vi "MAIN_PECT.vi"() -> ()   [LabVIEW 2018]
uses:
  <vilib>/DAQmx/read.llb/DAQmx Read (Analog 2D DBL NChan NSamp).vi
  <vilib>/Analysis/baseanly.llb/Mean (DBL).vi
  <vilib>/Instr/_visa.llb/VISA Configure Serial Port (Instr).vi
  <vilib>/DAQmx/create/channels.llb/DAQmx Create Channel (AI-Voltage-Basic).vi
  <vilib>/DAQmx/configure/timing.llb/DAQmx Timing (Sample Clock).vi
  <vilib>/DAQmx/configure/trigger.llb/DAQmx Start Trigger (Digital Edge).vi
  <vilib>/DAQmx/miscellaneous.llb/DAQmx Fill In Error Info.vi
  <resource>/objmgr/daqmx.rc
  <vilib>/Analysis/NI_AALBase.lvlib
  <vilib>/Platform/NI_3dgraph.lvlib
panel:
  out "Enum":T1(ring)=enum."Wait X"
  out "Current  Position (mm)":dbl=34.0
  out "Numeric":dbl=53.0
  in  "3D Surface":refnum<k7>(container)
  out "Feature extraction scan":dbl[](graph)=[0.08283467438816226, 0.08315021104927388, 0.08279539001624267, 0.08264303586690222, 0.08270737694574541, 0.08275255148264649, 0.08273400780940561, 0.08285927976479214, 0.08269226561515775, 0.08297621309518552, 0.08311167850920542, 0.08274828411115004, 0.08283507475884443, 0.08288811917638333, 0.08284021281644091, 0.08265273310686665, 0.082873404050702, 0.08252929871145775, 0.08289438074272544, 0.08328077996201763, 0.082870445586509, 0.08280965226600595, 0.08297444941499994, 0.08288058058223531, 0.08286124313516094, 0.08284469301402564, 0.083066551569298, 0.08282839970840086, 0.08295066176596085, 0.08313066697548752, 0.08296193038583091, 0.08281760657720119, 0.08275185969129775, 0.0830021575495491, 0.08289519151448965, 0.08270942154189498, 0.08314587726689038, 0.08300520769005512, 0.08316588069373743, 0.08268431002182852, 0.08284144737975019, 0.08280888249300979, 0.08277531905033915, 0.08291205402335713, 0.08302780379458881, 0.08284349413031018, 0.08272722568614103, 0.08294041368027252, 0.08290046841469481, 0.08300386096775844, 0.08306896615572697, 0.08269688952804832, 0.08275967850911117, 0.08263417478426685, 0.08279623232481706, 0.08272915933307569, 0.08286824410754713, 0.08291091733726794, 0.0830296712620475, 0.08266577930171704, 0.08258683375256373, 0.08276733860182627, 0.08282634908830305, 0.08298619981585892, 0.0828967582780724, 0.08282850993163872, 0.08273475855683762, 0.082968978472369, 0.0829109484443218, 0.0825587351950988, 0.08283584901550614, 0.08287979050131826, 0.08268241229465044, 0.08277735726888424, 0.08256618170984673, 0.08284253191870816, 0.08275059580850669, 0.08290221877356678, 0.08312313437093057, 0.0831193939376253, 0.08297293429910735, 0.08295049977967987, 0.08297761508701938, 0.08282735150019817, 0.0831591264906493, 0.08295251198394006, 0.08302823676291486, 0.08296307164975165, 0.08249046862995961, 0.08231989615770464, 0.08138645179421407, 0.07945694677113982, 0.07933082551380949, 0.08029170332009304, 0.08139752467180725, 0.08244302749015182, 0.08257548202947437, 0.08253717111330304, 0.0829704375877119, 0.08287075930532974, 0.08268538709012521, 0.08312089775665858, 0.08317847119013734, 0.0830002175397772, 0.082882772850329, 0.08311676213140336, 0.08291783582333187, 0.0829506193255121, 0.08276986520948888, 0.08300046343378967, 0.08275137325508078, 0.08277619485982919, 0.0828156000102155, 0.08269641985397105, 0.08263873798983143, 0.08270377967400899, 0.08291552507873104, 0.08270508332182003, 0.08289923248519893, 0.08282877191228727]
  in  "Cursor":bool=TRUE
  out "Completed":bool
  out "Acquire":bool
  in  "Step X":dbl=0.5
  in  "Freq_Sampling_SizeX_SizeY":dbl[](array[numeric])=[300.0, 100000.0]
  in  "Direction (+)":string="-"
  in  "X - length":dbl=60.0
  in  "Step Y":dbl=0.5
  in  "Y - length":dbl=60.0
  out "Start Pos Y":dbl
  out "Start Pos X":dbl
  in  "Scan":bool=TRUE
  in  "Motor only":bool
  out "Waveform Chart 2":dbl(graph)=0.08264330967693855
  in  "Offset":bool
  in  "Gate 2":dbl=25.0
  in  "Gate 1":dbl
  out "Backdata":dbl
  in  "Backdata":bool
  in  "Frame Avr.":i32=10
  in  "Digital Start Trigger Edge":i32(ring)=10280 caption="Edge" items=["Rising"=10280, "Falling"=10171]
  in  "Digital Start Trigger Source":tag="/Dev3/PFI0" caption="Trigger"
  in  "Move Dis(mm)":dbl=100.0
  out "Y Current.Pos(mm)":dbl=4.5 format="%#_4g"
  in  "COM Y":refnum<visa-resource-name>="COM3"
  in  "Multiplier":dbl=10.0
  in  "Travel per Pulse (mm)":dbl=0.004
  out "X Current.Pos(mm)":dbl=33.356 format="%#_4g"
  in  "Flow control":u16(ring) items=["None", "XON/XOFF", "RTS/CTS", "XON/XOFF & RTS/CTS", "DTR/DSR", "XON/XOFF & DTR/DSR"]
  in  "Stop bits":u16(ring)=10 items=["1.0"=10, "1.5"=15, "2.0"=20]
  in  "Speed (mm/s)":dbl=3.0
  in  "Stop":bool
  in  "Home":bool
  in  "Backward":bool
  in  "Left":bool
  in  "Forward":bool
  in  "Right":bool
  in  "Exit":bool
  in  "Parity":dbl
  in  "Data bits":u16=8 min=5 max=8 step=1
  in  "Baud Rate":u32=9600
  in  "COM X":refnum<visa-resource-name>="COM4"
  out "Waveform Graph 2":dbl[][](graph)=[[0.013601434298277221, 0.08376748657539852, 0.10555538260692392, 0.09988279438437878, 0.10291247214781425, 0.11561133460895198, 0.11364526707076025, 0.1047818478966451, 0.1184476286984939, 0.11196927511842217, 0.10416946617730119, 0.11116350971762164, 0.11264611793148685, 0.10397608257206907, 0.10935859528632208, 0.11171143016114275, 0.11361303649046076, 0.10852059925027957, 0.11586917952203521, 0.1124205037193586, 0.10584545813755739, 0.10919744219139764, 0.11280727102984134, 0.10397608256605081, 0.11080897297082777, 0.111066817844625, 0.11383865080705668, 0.10810160124557855, 0.11316180785941188, 0.11232381178111188, 0.10584545814989085, 0.10997097694527913, 0.11464441610483356, 0.10510415409350957, 0.11271057919576397, 0.11200150570035368, 0.11048666681159183, 0.10774706448063742, 0.11206596695446602, 0.11032551365379104, 0.10336370079032715, 0.10980982388310886, 0.11554687331452282, 0.10855282989125889, 0.1136774976544753, 0.11335519151887692, 0.10945528709246041, 0.10803714001130564, 0.11016436061280914, 0.10926190340085944, 0.09843241667361965, 0.11129243219726545, 0.11802863066881217, 0.10813383190229638, 0.11158250773738898, 0.11773855507696329, 0.10777929514448825, 0.10771483386556273, 0.1119370444031454, 0.1106478198754941, 0.09943156577112659, 0.11448326307988417, 0.11715840405452091, 0.10600661130849598, 0.11264611798894486, 0.11770632446719906, 0.10674791544461082, 0.10723137460757921, 0.11432210997511645, 0.11161473830411259, 0.10133317204675463, 0.11467664676291349, 0.11957570018781452, 0.10558761331160751, 0.10890736659450233, 0.1153212590005039, 0.10700576038234985, 0.10436284984003283, 0.11509564479684438, 0.11661048364039184, 0.10249347419312219, 0.11383865078746372, 0.12057484923885912, 0.10497523162681976, 0.10703799090530461, 0.11480556919139581, 0.10520084593006562, 0.10384716002193348, 0.11419318748956753, 0.1157724876889634, 0.10545869077007768, 0.11522456723740233, 0.12221861059120405, 0.10861729104683968, 0.10439508050894415, 0.11348411399724478, 0.10658676239523164, 0.10703799096366998, 0.11348411394953914, 0.11483779983544758, 0.105748766286294, 0.11364526710593634, 0.12089715535436718, 0.10842390737397982, 0.10358931516306184, 0.11351634464482596, 0.10839167680425396, 0.10974536256547154, 0.11428987936827059, 0.11506341408623584, 0.10433061916843969, 0.11184035263979672, 0.11625594670038104, 0.10439508050888772, 0.10758591145457821, 0.11699725106811235, 0.11097012602935477, 0.11077674228063383, 0.11690055921882556, 0.1119370443655943, 0.10391162120758887, 0.11100235666681757, 0.11377418946627674, 0.10313808654861531, 0.10668345422161463, 0.12063931049392565, 0.11213042817800026, 0.11032551358979706, 0.11748071025092614, 0.11171143006960613, 0.10600661125928526, 0.10723137464977092, 0.11551464274992203, 0.1009141740623463, 0.11000320758245671, 0.12205745752266203, 0.1106800504822431, 0.1088751360032324, 0.12070377174855577, 0.10806937058012958, 0.10568430507660669, 0.10961644014725073, 0.11532125899335136, 0.10084971283493516, 0.1129684241513111, 0.1211872309349945, 0.11055112802413684, 0.10613553370420262, 0.11964016142031346, 0.10674791538099922, 0.10371823751735168, 0.11245273434937711, 0.11722286520589442, 0.10578099696801421, 0.11164696886759451, 0.12228307187689273, 0.11013213004518332, 0.10204224553504146, 0.11673940609854719, 0.10819829306708265, 0.10265462716988191, 0.11470887734845048, 0.12099384718962294, 0.10652230113094655, 0.1138064201020185, 0.12221861065750776, 0.1102610524735794, 0.08334848852242217, -0.058788534635624334, -0.11989779045978155, -0.14017085139642654, -0.1336280352805537, -0.12801990704400926, -0.14600459383486838, -0.13801139971037607, -0.1311462772922099, -0.14107330877412233, -0.14967888479881436, -0.13733455662936145, -0.14065431057136318, -0.14774504739847086, -0.13475610701189997, -0.13156527533589288, -0.14858304359243135, -0.14136338429903875, -0.13079174085124246, -0.14258814791681923, -0.15029126661441775, -0.12972812989040167, -0.14197576622098812, -0.14484429156186746, -0.13362803512777408, -0.13166196732019605, -0.15132264646204385, -0.14171792120587728, -0.13240327180667855, -0.14858304358489416, -0.14671366757571636, -0.1247968448647718, -0.14242699487971355, -0.1427493011356822, -0.13224211836195246, -0.1359808705608181, -0.15035572777198442, -0.14719712698964665, -0.13140412236860619, -0.15103257084729058, -0.14371621972211224, -0.1263116841459282, -0.1403642349991318, -0.1424592254369844, -0.12889013376813427, -0.14191130491799478, -0.14809958426479436, -0.14677812889654474, -0.13111404665168178, -0.15177387515944252, -0.13936508580925389, -0.12669845160863982, -0.1428459928421259, -0.14700374310609157, -0.13037274236425173, -0.1458756714525446, -0.14684259002493194, -0.14361952793272406, -0.13104958540060116, -0.14677812876602267, -0.1381080916109839, -0.13108181602987884, -0.14233030290956655, -0.1491954254599751, -0.1326611164851572, -0.144167448547146, -0.15051688097972826, -0.14023531251808827, -0.12885790319962048, -0.14274930102339384, -0.1415245375090149, -0.13111404663251974, -0.14336168282353604, -0.1502590359852162, -0.13688332796086422, -0.14091215576342137, -0.15112926275912902, -0.14004192882973127, -0.12808436827914507, -0.14181461295870892, -0.1407510025200201, -0.1309206629510732, -0.14339391351034778, -0.15454570867573808, -0.13913947146510475, -0.13817255274502313, -0.15190279768123222, -0.13620648496892968, -0.1339825719914834, -0.14303937657753946, -0.14220138051954856, -0.13330572894558984, -0.14107330876402224, -0.15322425317405103, -0.13527179685661722, -0.13926839391275525, -0.1468425900501376, -0.13765686282695927, -0.13395034137824646, -0.14913096409414178, -0.14220138056245094, -0.13610979309633864, -0.1428459929306679, -0.1514193383764275, -0.13362803506894924, -0.13694778927852186, -0.14529552018613665, -0.13627094604099171, -0.13662548295342475, -0.14664920627251926, -0.14703597378395564, -0.13720563421577722, -0.14407075652821602, -0.14787396992634924, -0.13565856431412787, -0.1359808705794155, -0.1445864464810054, -0.1380436302301929, -0.14162122931720006, -0.14307160730830817, -0.1510970321115987, -0.1368188666778612, -0.14323276036380136, -0.14626243883029288, -0.13652879115001798, -0.13301565343259897, -0.14681035935072898, -0.1381080914941658, -0.14123446183340477, -0.14071877196186522, -0.1513871077424996, -0.13543294994218183, -0.14213691925180744], [0.5037481552143733, 0.4782859739390544, 0.5250203570724526, 0.49504589076072747, 0.4966574212176529, 0.48118672878275026, 0.534367233585223, 0.4808644226891975, 0.5098719709209371, 0.5150288683453328, 0.5095496648315279, 0.477963667845071, 0.5263095814212335, 0.4956905029436372, 0.49407897248601346, 0.4808644226891975, 0.5179296231414922, 0.483442871436285, 0.5024589308529928, 0.5166403987880918, 0.5130950318125386, 0.48569901408749055, 0.5188965414060729, 0.5024589308529928, 0.49053360547513025, 0.4911782176593487, 0.5056819917550686, 0.48569901408749055, 0.5018143186720267, 0.5134173379014503, 0.5085827465630276, 0.4937566663943488, 0.5140619500791384, 0.5063266039349343, 0.49085591156726294, 0.503425849124097, 0.503425849124097, 0.4889220750137619, 0.5002027882188058, 0.5121281135455329, 0.5014920125814748, 0.5005250943095422, 0.510194277010301, 0.5105165830996194, 0.4869882384585658, 0.5140619500791384, 0.5018143186720267, 0.49407897248601346, 0.4966574212176529, 0.5185742353179239, 0.4934343603026375, 0.5043927673947882, 0.5031035430337749, 0.5098719709209371, 0.4892443811061296, 0.5188965414060729, 0.5027812369434068, 0.4998804821280232, 0.4985912577644308, 0.5304995605499158, 0.4882774628288851, 0.5011697064908767, 0.5060042978450243, 0.5050373795750199, 0.48215364706312236, 0.5240534388104038, 0.5005250943095422, 0.5014920125814748, 0.49085591156726294, 0.5424248857221113, 0.48795515673637607, 0.5037481552143733, 0.504715073484927, 0.5085827465630276, 0.47860828003298983, 0.523086520547957, 0.5008474004002325, 0.5014920125814748, 0.480542116595597, 0.541457967467102, 0.4892443811061296, 0.5002027882188058, 0.5105165830996194, 0.5130950318125386, 0.47602983128016196, 0.5234088266354835, 0.5040704613046038, 0.4985912577644308, 0.47538521909147413, 0.5308218666364309, 0.4892443811061296, 0.5018143186720267, 0.5118058074564408, 0.5234088266354835, 0.47506291299705794, 0.5205080718461484, 0.510194277010301, 0.49472358466920274, 0.4776413617510396, 0.5166403987880918, 0.4892443811061296, 0.4995581760371945, 0.5118058074564408, 0.5243757448977976, 0.4895666871984503, 0.5150288683453328, 0.5166403987880918, 0.49021129938295055, 0.4892443811061296, 0.5095496648315279, 0.49053360547513025, 0.49504589076072747, 0.5150288683453328, 0.5159957866111228, 0.4969797273088985, 0.5072935222043906, 0.5179296231414922, 0.4911782176593487, 0.4989135638553983, 0.5092273587420731, 0.4969797273088985, 0.4937566663943488, 0.5124504196345799, 0.5095496648315279, 0.4969797273088985, 0.5037481552143733, 0.5179296231414922, 0.4921451359353248, 0.510194277010301, 0.5072935222043906, 0.5040704613046038, 0.4924674420272231, 0.5243757448977976, 0.4989135638553983, 0.4973020334000977, 0.5005250943095422, 0.516962704876509, 0.48795515673637607, 0.516962704876509, 0.5076158282941181, 0.5060042978450243, 0.4953681968522056, 0.5363010701005323, 0.4976243394912505, 0.4918228298433796, 0.5011697064908767, 0.5159957866111228, 0.47860828003298983, 0.5201857657582224, 0.5069712161146175, 0.5056819917550686, 0.48569901408749055, 0.5411356613820134, 0.49504589076072747, 0.49826895167341706, 0.5037481552143733, 0.5185742353179239, 0.47602983128016196, 0.5227642144603862, 0.5082604404734367, 0.5040704613046038, 0.4718398520502395, 0.5356564579289357, 0.49407897248601346, 0.4969797273088985, 0.5072935222043906, 0.5275988057693101, -0.5192517469977762, -0.4812195963717544, -0.4818642090794271, -0.49959105873960724, -0.5337555337266507, -0.47348424391910443, -0.5070041050757489, -0.5031364287179863, -0.48605419169165304, -0.46832734232432, -0.5169956024191665, -0.48218651543345337, -0.4818642090794271, -0.5002356714617954, -0.5256978744002724, -0.48315343449629206, -0.5070041050757489, -0.5073264114397315, -0.48412035356027106, -0.47090579311768965, -0.5060371859845731, -0.487343417115113, -0.4763850010803293, -0.504425654168518, -0.5115163941832249, -0.4886326425406057, -0.5012025905460384, -0.5140948451131326, -0.4847649662702243, -0.4802526773111943, -0.504425654168518, -0.4937895442629384, -0.4776742264885969, -0.5047479605314721, -0.5002356714617954, -0.4895995616110602, -0.49540107605786016, -0.5131279260134487, -0.48315343449629206, -0.486698804403129, -0.5053925732577655, -0.4989464460179313, -0.47574038837695243, -0.5070041050757489, -0.4950787696986205, -0.48605419169165304, -0.49056648068265996, -0.5157063769485245, -0.46993887406923396, -0.4944341569805242, -0.5095825559912142, -0.5037810414429954, -0.47509577567408007, -0.5157063769485245, -0.4886326425406057, -0.48605419169165304, -0.4937895442629384, -0.5182848278918804, -0.4593027646106859, -0.5008802841844959, -0.5076487178038427, -0.4999133651006372, -0.47864114554612325, -0.5173179087871507, -0.4883103361840418, -0.48927725525411486, -0.4947564633395085, -0.5282763253758406, -0.46284813441505984, -0.49959105873960724, -0.5050702668945546, -0.49797952693637737, -0.47058348676807876, -0.5179625215235075, -0.4883103361840418, -0.4889549488972967, -0.49217801247120607, -0.5373009038561416, -0.4715504058172886, -0.49959105873960724, -0.5063594923481698, -0.49121109339769625, -0.4673604232788777, -0.5153840705811875, -0.48992186796813286, -0.4895995616110602, -0.4950787696986205, -0.5340778401014041, -0.486698804403129, -0.4989464460179313, -0.5070041050757489, -0.4918557061132421, -0.46510427884390065, -0.5099048623562269, -0.49701260785597473, -0.48379804720548464, -0.4989464460179313, -0.5247309552865832, -0.49056648068265996, -0.4950787696986205, -0.5082933305324514, -0.49411185062166746, -0.4715504058172886, -0.5053925732577655, -0.5021695096314351, -0.48347574085082495, -0.49797952693637737, -0.5111940878175674, -0.4944341569805242, -0.48992186796813286, -0.5082933305324514, -0.4973349142159811, -0.4818642090794271, -0.5060371859845731, -0.5082933305324514, -0.48154190272552744, -0.4999133651006372, -0.5024918159934906, -0.48927725525411486, -0.4895995616110602, -0.5105494750866392, -0.4889549488972967, -0.4934672379043369, -0.5041033478056925, -0.5082933305324514, -0.48702111075905746, -0.49926875237870527, -0.49862413965728536, -0.49153339975540544, -0.4854095789806849, -0.5079710241680827, -0.4879880298276051, -0.49411185062166746]]
  in  "length":i32
  in  "Start index":i32
  in  "Path":path
  in  "Name File":string
  in  "SAVE ?":bool
  in  "Number of Samples":i32=400
  in  "Sample Rate":dbl=100000.0
  in  "Sample Clock Source":tag="OnboardClock"
  in  "Terminal Configuration":i32(ring)=10083 items=["default"=-1, "RSE"=10083, "NRSE"=10078, "Differential"=10106, "Pseudodifferential"=12529]
  in  "Max Voltage":dbl=10.0
  in  "Min Voltage":dbl=-10.0
  in  "Physical Channel":tag="Dev3/ai1:2"
  out "Actual Sample Rate":dbl=100000.0 format="%0.2f"
  # "Graph"
  # "Channel Settings"
  # "Control Program"
  # "Timing Settings"
  # "Saving Data Settings"
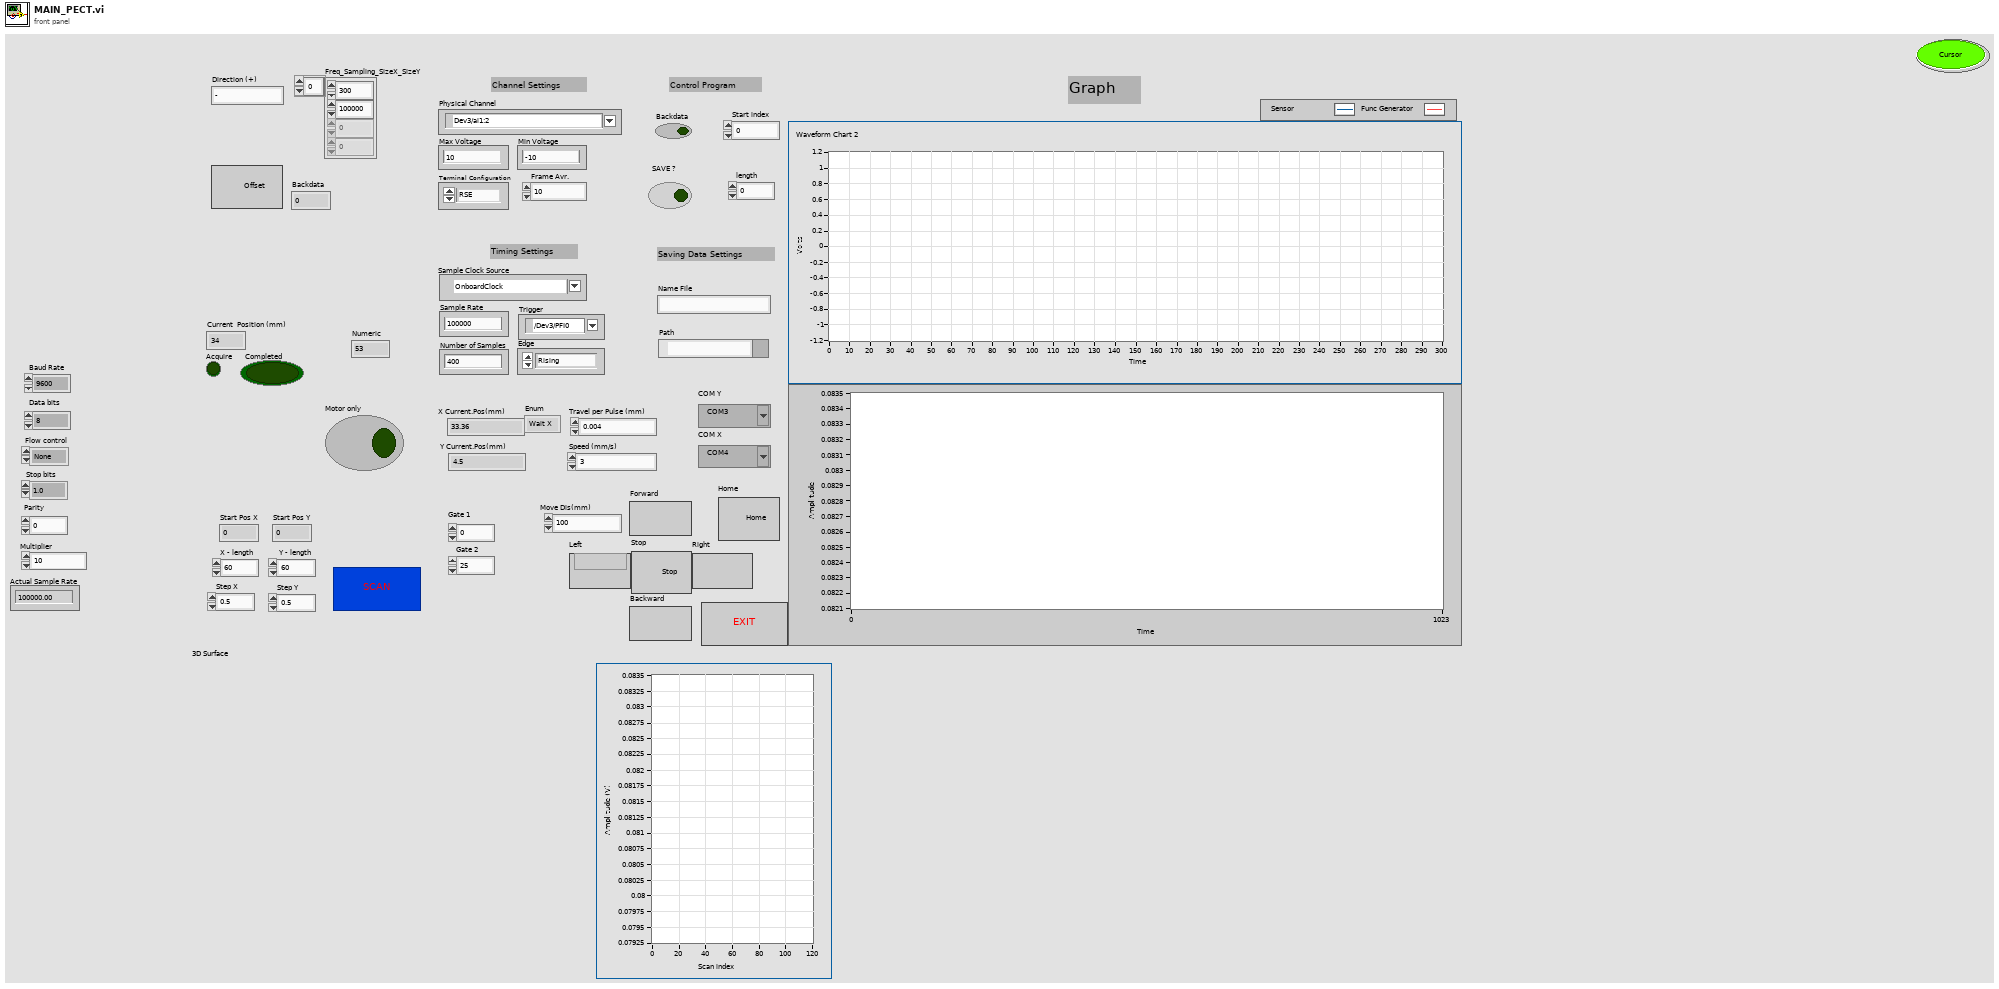
[diagram p1: front panel]
types:
  T1 = enum16{"No Scan", "Move X", "Wait X", "Move Y", "Wait Y"}
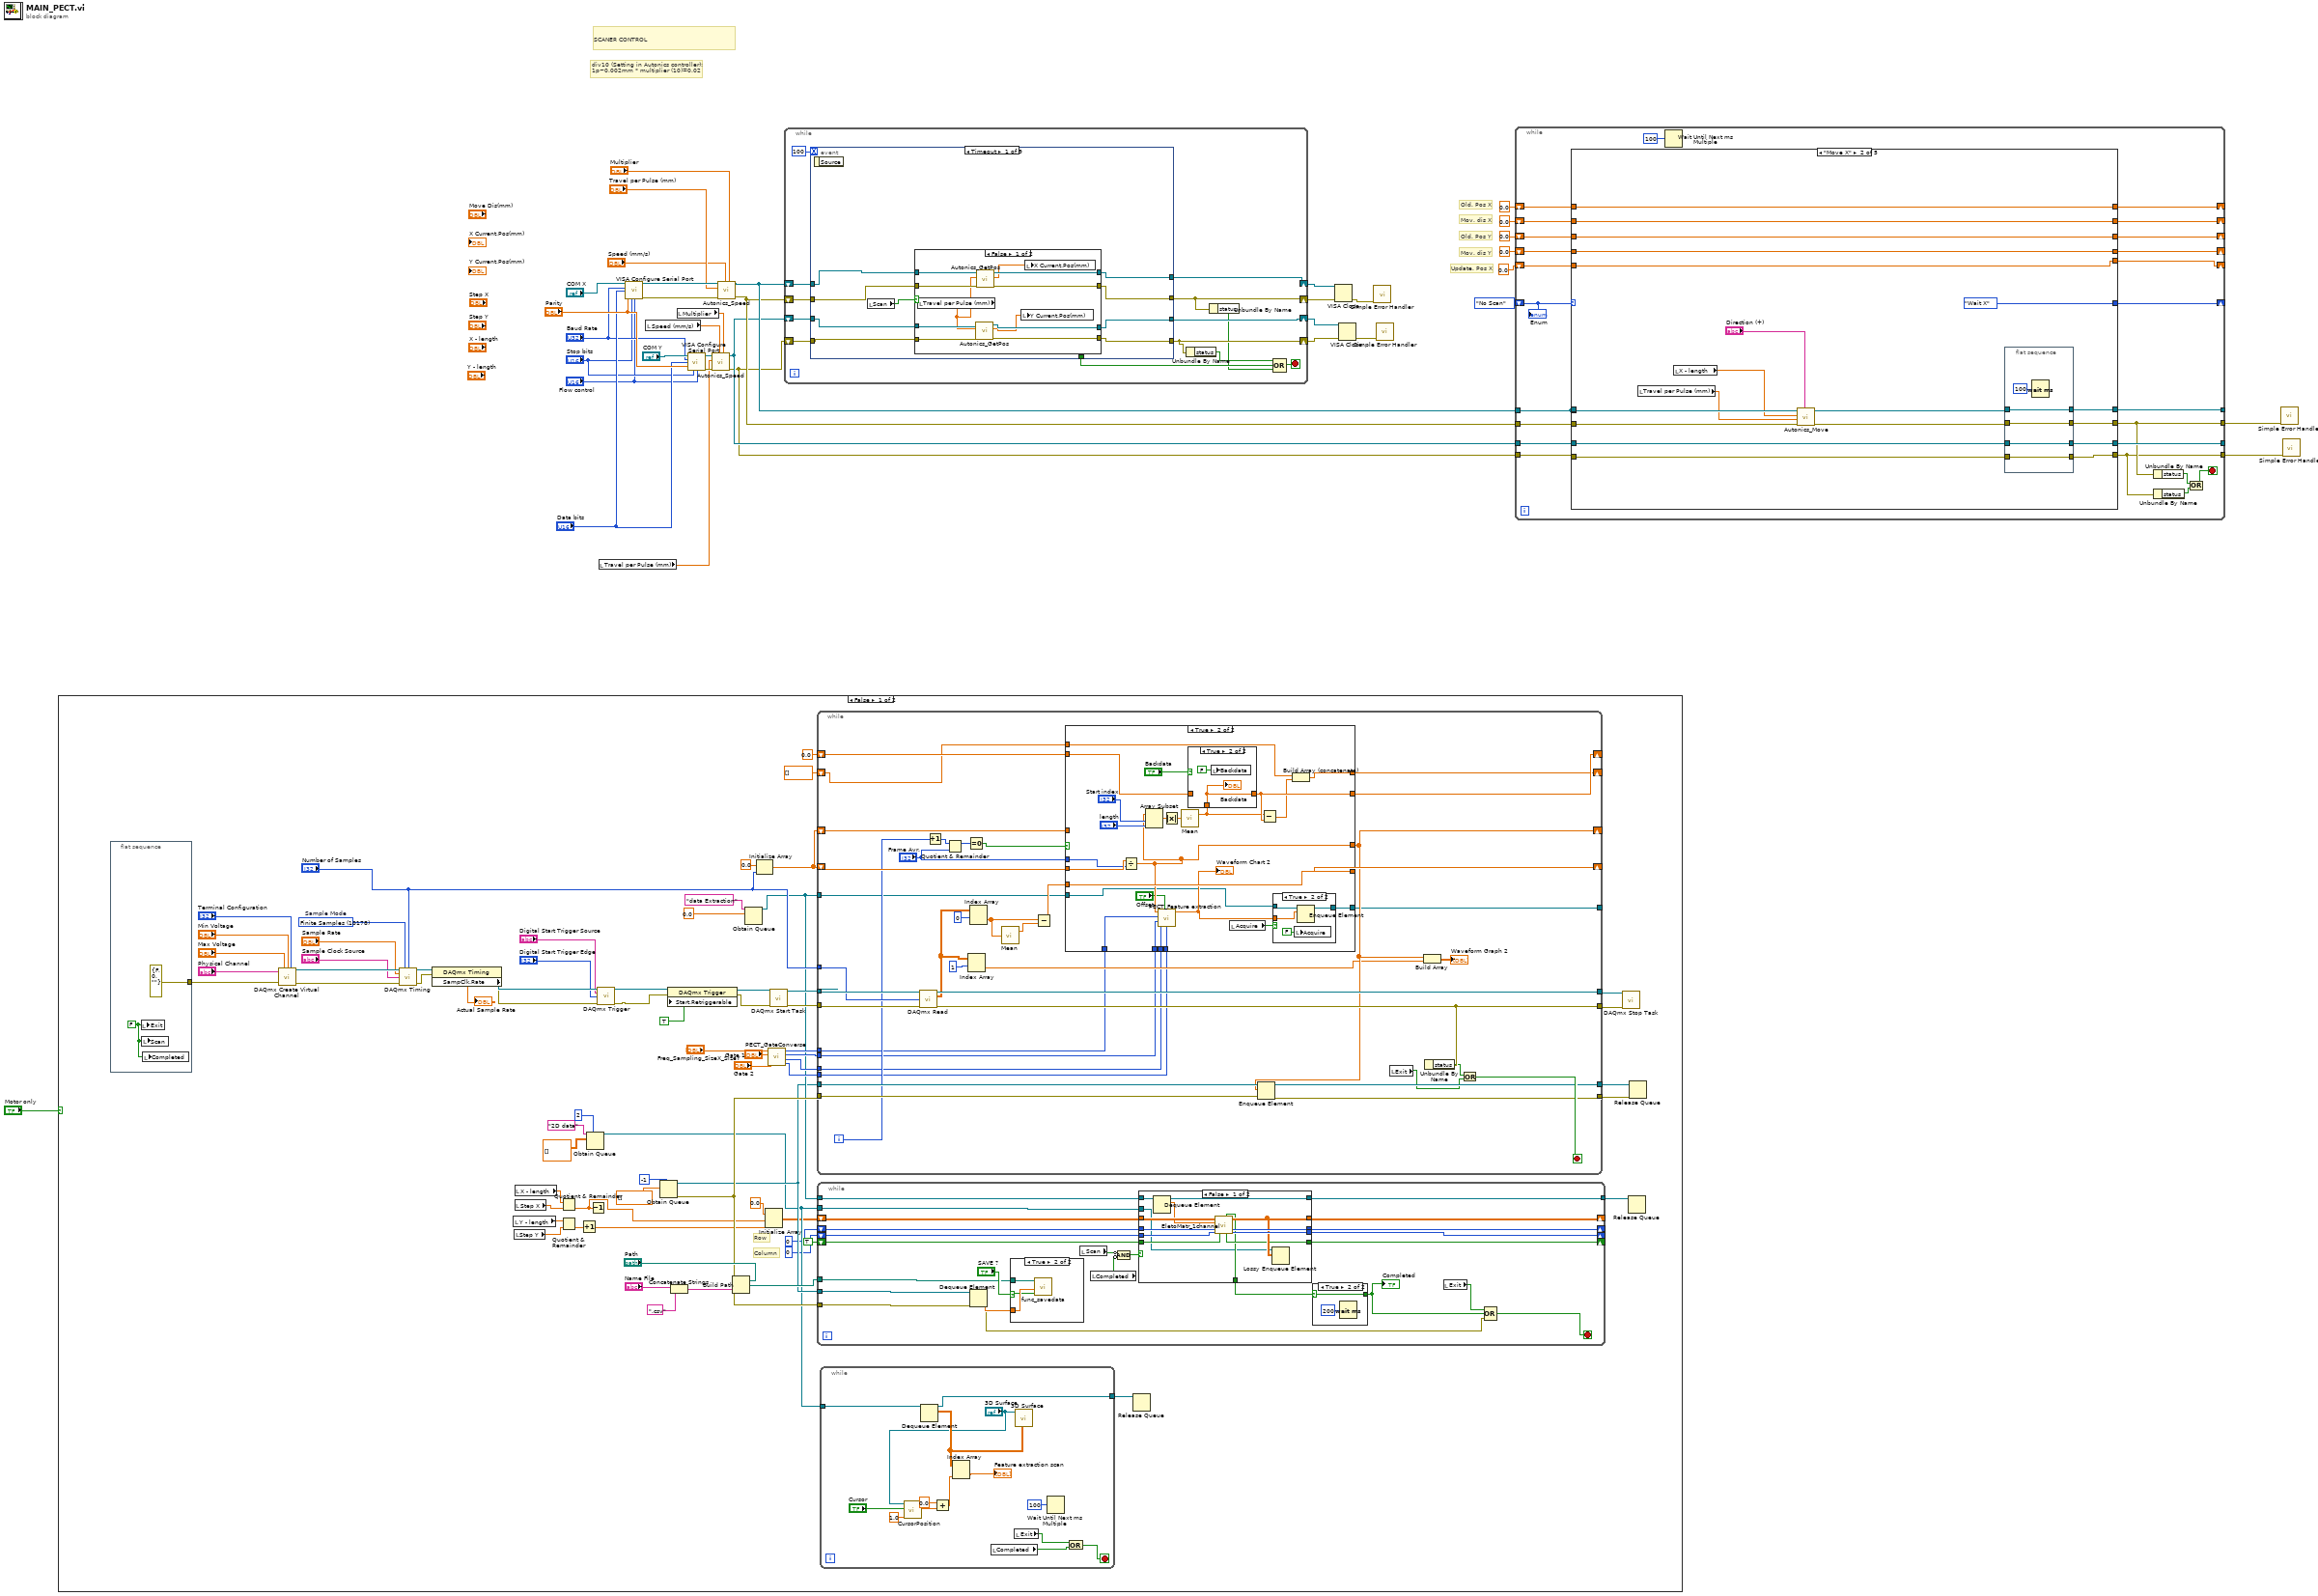
[diagram p0: block diagram]
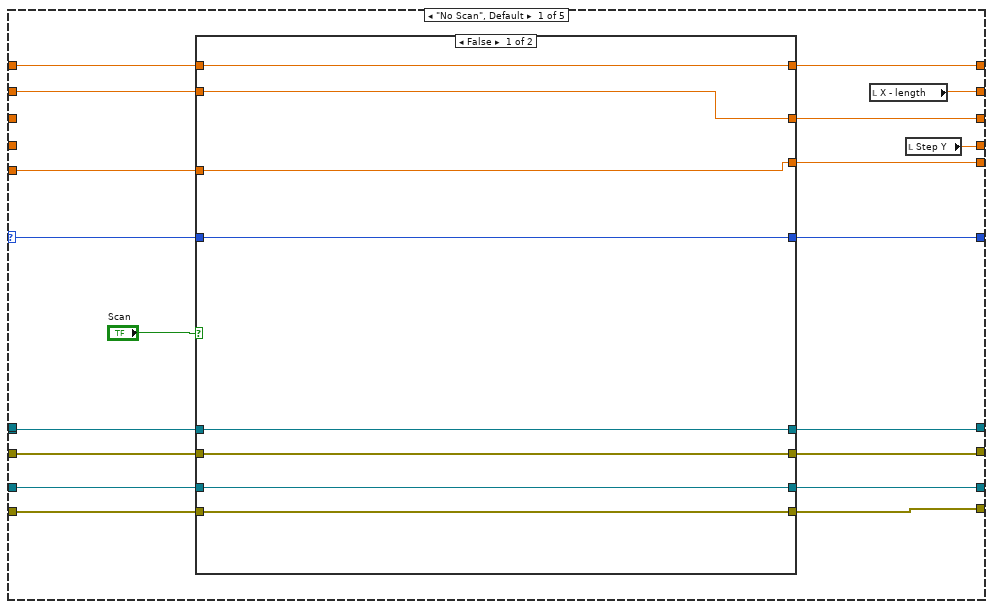
[diagram p2: hidden frame]
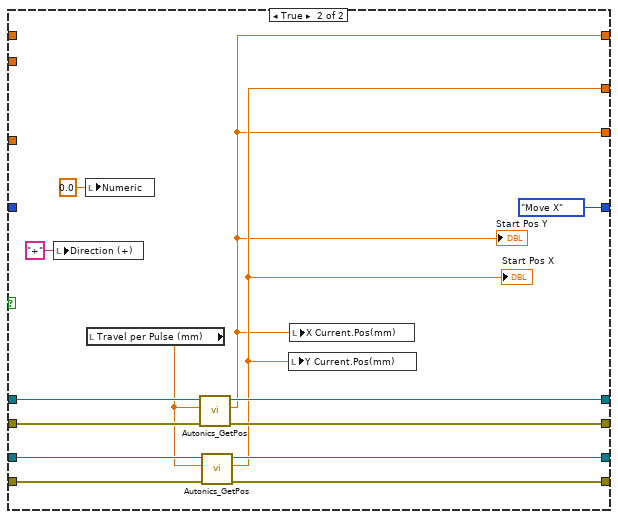
[diagram p3: hidden frame]
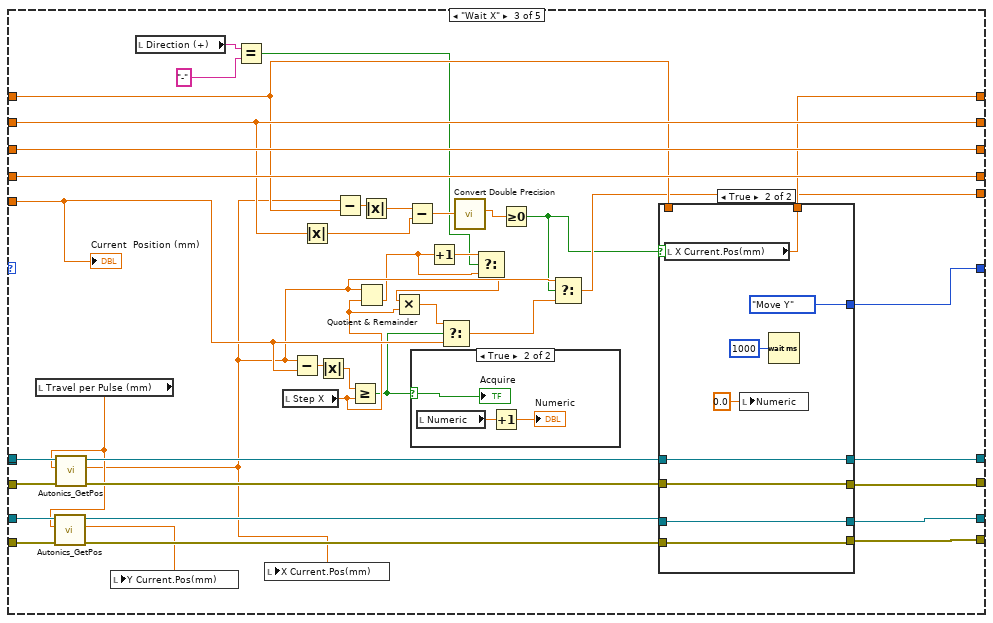
[diagram p4: hidden frame]
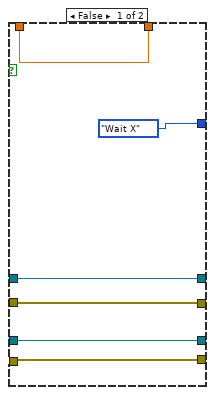
[diagram p6: hidden frame]
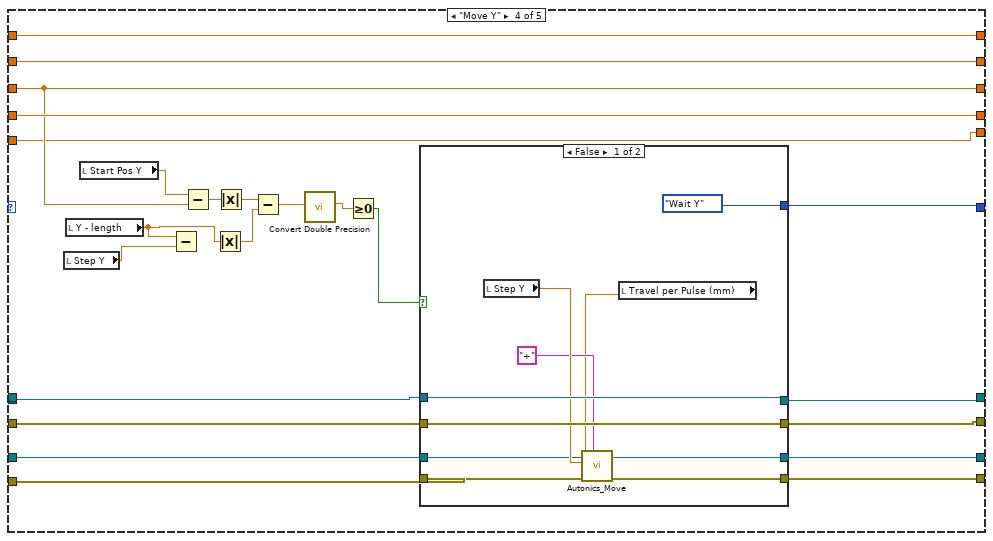
[diagram p7: hidden frame]
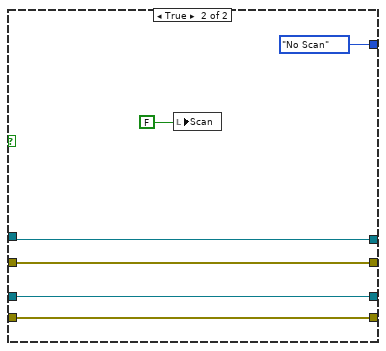
[diagram p8: hidden frame]
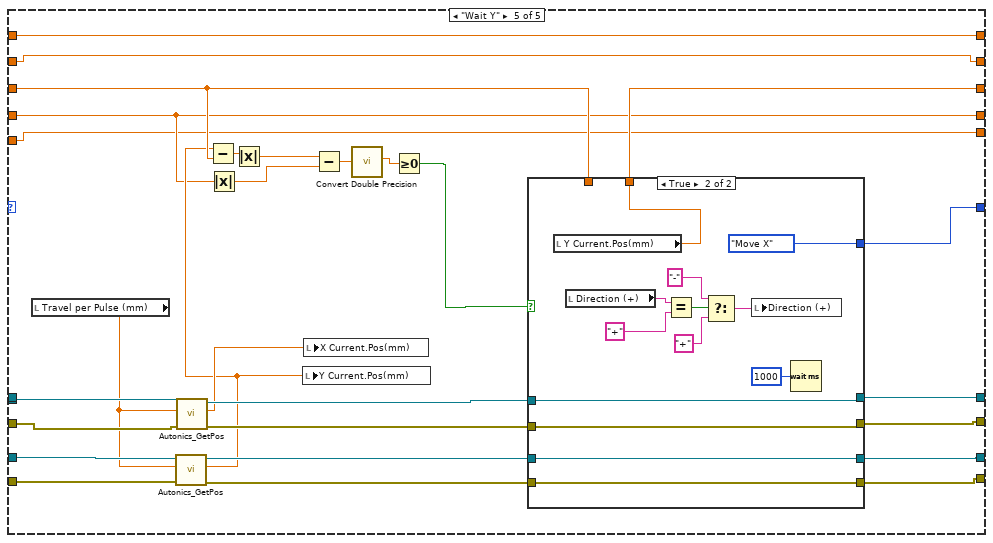
[diagram p9: hidden frame]
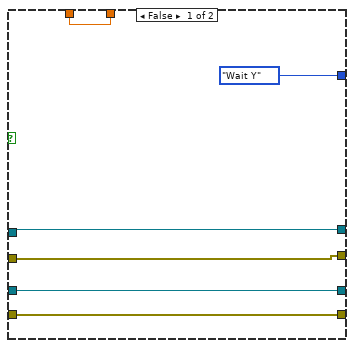
[diagram p10: hidden frame]
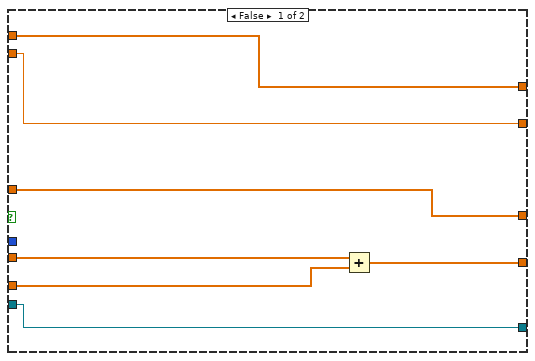
[diagram p14: hidden frame]
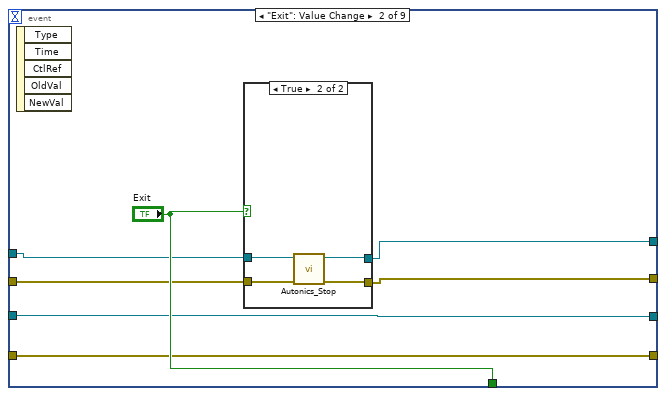
[diagram p19: hidden frame]
diagram:
  # "Update. Pos X"
  # "Mov. dis Y"
  # "Old. Pos Y"
  # "Mov. dis X"
  # "Old. Pos X"
  # "div10 (Setting in Autonics controller):\n1p~0.002mm * multiplier (10)=0.02"
  # "SCANER CONTROL"
  n1 = case shown="False" "Motor only" {
    frame False {
      w104 = 10178 items=["Finite Samples"=10178, "Continuous Samples"=10123, "Hardware Timed Single Point"=12522]  # Sample Mode
      # "Column"
      # "Row"
      n2 = flat-sequence {
        tunnel: [errorcluster {"status"=FALSE, "code"=0, "source"=""} ("error in")] -> w74
        frame #0 {
          w169 = FALSE ("Exit")
          n3 = local write "Exit"(w169) -> ()
          n4 = local write "Scan"(w169) -> ()
          n5 = local write "Completed"(w169) -> ()
        }
      }
      n6 = call-poly <vilib>:"DAQmx Create Virtual Channel.vi"("maximum value"="Max Voltage", "minimum value"="Min Voltage", "input terminal configuration"="Terminal Configuration", "physical channels"="Physical Channel", "error in"=w74) -> ("task out"=w102:refnum<k21>, "error out"=w103:errorcluster)  [unwired: 9 in]
      n7 = call-poly <vilib>:"DAQmx Timing.vi"("task/channels in"=w102, "sample mode"=w104, "samples per channel"="Number of Samples", "rate"="Sample Rate", "source"="Sample Clock Source", "error in"=w103) -> ("task out"=w106:refnum<k21>, "error out"=w105:errorcluster)  [unwired: 8 in]
      n8 = property class="DAQmx Timing"(reference=w106, error in=w105) -> (reference out=w95:refnum<k21>, error out=w94:errorcluster, "SampClk.Rate"=→"Actual Sample Rate":dbl)
      n9 = local read "Y - length"() -> (w54:dbl)
      n10 = local read "Step Y"() -> (w53:dbl)
      n11 = local read "X - length"() -> (w56:dbl)
      n12 = local read "Step X"() -> (w55:dbl)
      n13 = Quotient & Remainder(x=w56, y=w55) -> (floor(x/y)=w37:dbl)  [unwired: 1 out]
      n14 = Quotient & Remainder(x=w54, y=w53) -> (floor(x/y)=w52:dbl)  [unwired: 1 out]
      n15 = Increment(x=w52) -> (x+1=w45:dbl)
      n16 = Obtain Queue(max queue size (-1, unlimited)=2 ("최대 큐 크기(-1,제한없음)"), name (unnamed)="2D data", element data type=dbl[][] [] ("initialized array")) -> (queue out=w46:refnum<queue>)  [unwired: 2 in, 2 out]
      n17 = Decrement(x=w37) -> ()  [unwired: 1 out]
      n18 = call-poly <vilib>:"DAQmx Trigger.vi"("task/channels in"=w95, "source"="Digital Start Trigger Source", "edge"="Digital Start Trigger Edge", "error in"=w94) -> ("task out"=w72:refnum<k21>, "error out"=w71:errorcluster)  [unwired: 10 in]
      n19 = Obtain Queue(max queue size (-1, unlimited)=-1, element data type=dbl[] [] ("Radar output")) -> (queue out=w47:refnum<queue>, error out=w81:errorcluster)  [unwired: 3 in, 1 out]
      n20 = property class="DAQmx Trigger"(reference=w72, error in=w71, "Start.Retriggerable"=TRUE) -> (reference out=w70:refnum<k21>, error out=w69:errorcluster)
      n21 = Concatenate Strings("Name File", ".csv" ("string")) -> (w87:string)
      n22 = Build Path(base path="Path", name or relative path=w87) -> (appended path=w85:path)
      n23 = Obtain Queue(name (unnamed)="data Extraction", element data type=0.0) -> (queue out=w51:refnum<queue>)  [unwired: 3 in, 2 out]
      n24 = Initialize Array(0.0 ("element"), "Number of Samples") -> (w79:dbl[])
      n25 = Initialize Array(0.0 ("element"), w37, w45) -> (w43:dbl[][])
      n26 = call "PECT_GateConverse.vi"("Gate 2"="Gate 2", "Gate 1"="Gate 1", "Freq_Sampling_SizeX_SizeY"="Freq_Sampling_SizeX_SizeY") -> ("Length T/2"=w63:i32, "Length"=w64:i32, "Start 2"=w65:i32, "Start 1"=w66:i32)  [unwired: 5 in]
      n27 = call <vilib>:"DAQmx Start Task.vi"("task/channels in"=w70, "error in"=w69) -> ("task out"=w91:refnum<k21>, "error out"=w90:errorcluster)  [unwired: 12 in]
      n28 = while {
        tunnel: w91 -> [w209]
        tunnel: w90 -> [w208]
        tunnel: [w207] -> w93
        tunnel: [w206] -> w92
        tunnel: "Number of Samples" -> [w204]
        tunnel: w47 -> [w201]
        tunnel: w81 -> [w200]
        tunnel: [w182] -> w82
        shift-right: [w196] -> _
        shift-left: w79 -> [w198]
        shift-right: [w188] -> _
        shift-left: w79 -> [w191]
        tunnel: [w186] -> w76
        shift-right: [w183] -> _
        shift-left: 0.0 ("mean") -> [w184]
        shift-right: [w180] -> _
        shift-left: dbl[] [] -> [w179]
        tunnel: w66 -> [w178]
        tunnel: w65 -> [w177]
        tunnel: w64 -> [w176]
        tunnel: w63 -> [w175]
        tunnel: [w172] -> _
        tunnel: w51 -> [w171]
        i -> [w195]
        stop <- w202 stop-if-true
        n29 = call-poly <vilib>:"DAQmx Read.vi"("task/channels in"=w209, "number of samples per channel"=w204, "error in"=w208) -> ("task out"=w207:refnum<k21>, "data"=w174:dbl[][], "error out"=w206:errorcluster)  [unwired: 10 in]
        n30 = Increment(x=w195) -> (x+1=w194:i32)
        n31 = Quotient & Remainder(x=w194, y="Frame Avr.") -> (x-y*floor(x/y)=w193:i32)  [unwired: 1 out]
        n32 = Equal To 0?(x=w193) -> (x = 0?=w181:bool)
        n33 = Index Array(array=w174, index (row)=1) -> (element=w187:dbl[])  [unwired: 1 in]
        n34 = Index Array(array=w174, index (row)=0) -> (element=w190:dbl[])  [unwired: 1 in]
        n35 = call-poly <vilib>:"Mean.vi"("X"=w190) -> ("mean"=w199:dbl)  [unwired: 1 out]
        n36 = Subtract(x=w190, y=w199) -> (x-y=w197:dbl[])
        n37 = case shown="True" w181 {
          tunnel: w198 -> [w216 w240]
          tunnel: w197 -> [w215 w239]
          tunnel: [w214 w239] -> w196
          tunnel: "Frame Avr." -> [_ w232]
          tunnel: [w213 w227] -> w188
          tunnel: w191 -> [w213 _]
          tunnel: w184 -> [w212 w234]
          tunnel: [w212 w233] -> w183
          tunnel: [w211 w229] -> w180
          tunnel: w179 -> [w211 w230]
          tunnel: w178 -> [_ w226]
          tunnel: w177 -> [_ w225]
          tunnel: w176 -> [_ w224]
          tunnel: w175 -> [_ w223]
          tunnel: [w210 w219] -> w172
          tunnel: w171 -> [w210 w218]
          frame False {
            n38 = Add(x=w216, y=w215) -> (x+y=w214:dbl[])
          }
          frame True {
            n39 = Divide(x=w240, y=w232) -> (x/y=w227:dbl[])
            n40 = Array Subset(array=w227, index="Start index", length="length") -> (w236:dbl[])
            n41 = call "PECT_Feature extraction.vi"("Length T/2"=w223, "Offset"="Offset", "Length"=w224, "Start 2"=w225, "Start 1"=w226, "Pulse signal in"=w227) -> ("Feature extraction out"=w220:dbl)  [unwired: 5 in]
            "Waveform Chart 2" <- w220
            n42 = Absolute Value(x=w236) -> (abs(x)=w237:dbl[])
            n43 = call-poly <vilib>:"Mean.vi"("X"=w237) -> ("mean"=w231:dbl)  [unwired: 1 out]
            n44 = case shown="True" "Backdata" {
              tunnel: w231 -> [_ w248]
              tunnel: [w246 w248] -> w233
              tunnel: w234 -> [w246 _]
              frame False {
              }
              frame True {
                n45 = local write "Backdata"(FALSE ("Backdata")) -> ()
                "Backdata" <- w248
              }
            }
            n46 = local read "Acquire"() -> (w217:bool)
            n47 = Subtract(x=w231, y=w233) -> (x-y=w221:dbl)
            n48 = case shown="True" w217 {
              tunnel: w220 -> [_ w244]
              tunnel: [w241 w243] -> w219
              tunnel: w218 -> [w241 w242]
              frame False {
              }
              frame True {
                n49 = local write "Acquire"(FALSE ("Acquire")) -> ()
                n50 = Enqueue Element(queue=w242, element=w244) -> (queue out=w243:refnum<queue>)  [unwired: 2 in, 2 out]
              }
            }
            n51 = Build Array (concatenate)(w230, w221) -> (w229:dbl[])
          }
        }
        n52 = Enqueue Element(queue=w201, element=w188, error in (no error)=w200) -> (queue out=w186:refnum<queue>, error out=w182:errorcluster)  [unwired: 1 in, 1 out]
        n53 = local read "Exit"() -> (w185:bool)
        n54 = Build Array(w188, w187) -> (→"Waveform Graph 2":dbl[][])
        n55 = Unbundle By Name(w206) -> ("status"=w205:bool)
        n56 = Or(x=w205, y=w185) -> (x .or. y?=w202:bool)
      }
      n57 = while {
        tunnel: w81 -> [w127]
        tunnel: w47 -> [w128]
        tunnel: w85 -> [w129]
        shift-right: [w119] -> _
        shift-left: w43 -> [w124]
        tunnel: w51 -> [w125]
        shift-right: [w121] -> _
        shift-left: 0 -> [w123]
        shift-right: [w120] -> _
        shift-left: 0 -> [w122]
        shift-right: [w118] -> _
        shift-left: TRUE ("Output Direction") -> [w117]
        tunnel: w46 -> [w108]
        tunnel: [w107] -> w39
        stop <- w113 stop-if-true
        n58 = Dequeue Element(queue=w128, error in (no error)=w127) -> (element=w126:dbl[], error out=w115:errorcluster)  [unwired: 1 in, 2 out]
        n59 = case shown="True" "SAVE ?" {
          selector: "SAVE ?" -> [_ w152]
          tunnel: w126 -> [_ w153]
          tunnel: w129 -> [_ w154]
          frame False {
          }
          frame True {
            n60 = call "func_savedata.vi"("append to file? (new file:F)"=w152, "1D data"=w153, "file path (dialog if empty)"=w154) -> ()  [unwired: 9 in]
          }
        }
        n61 = local read "Scan"() -> (w110:bool)
        n62 = local read "Completed"() -> (w111:bool)
        n63 = Compound Arithmetic op=AND(invert w110, invert w111) -> (w109:bool)
        n64 = case shown="False" w109 {
          tunnel: w125 -> [w146 w147]
          tunnel: w124 -> [w145 w151]
          tunnel: w123 -> [w143 w150]
          tunnel: w122 -> [w142 w149]
          tunnel: [w141 w150] -> w121
          tunnel: [w140 w149] -> w120
          tunnel: [w139 w151] -> w119
          tunnel: [w138 w148] -> w118
          tunnel: w117 -> [w137 w148]
          tunnel: [w136 _] -> w116
          tunnel: w108 -> [w135 _]
          tunnel: [w134 w147] -> w107
          frame False {
            n65 = Dequeue Element(queue=w146) -> (queue out=w134:refnum<queue>, element=w144:dbl)  [unwired: 2 in, 2 out]
            n66 = call "EletoMatr_1channel.vi"("Input Array X"=w145, "Input data"=w144, "In Row"=w143, "In Column"=w142, "Input Direction"=w137) -> ("Completed"=w136:bool, "Out Array X"=w139:dbl[][], "Out Row"=w141:i32, "Output Direction"=w138:bool, "Out Column"=w140:i32)  [unwired: 6 in]
            n67 = Lossy Enqueue Element(queue=w135, element=w139) -> ()  [unwired: 1 in, 4 out]
          }
          frame True {
          }
        }
        n68 = case shown="True" w116 {
          selector: w116 -> [w131 w132]
          tunnel: [w131 w132] -> w114
          frame False {
          }
          frame True {
            n69 = Wait (ms)(milliseconds to wait=u32 200) -> ()  [unwired: 1 out]
          }
        }
        "Completed" <- w114
        n70 = local read "Exit"() -> (w112:bool)
        n71 = Compound Arithmetic op=OR(w112, w114, w115) -> (w113:bool)
      }
      n72 = while {
        tunnel: w46 -> [w157]
        tunnel: [w156] -> w38
        stop <- w158 stop-if-true
        n73 = call "CursorPosition.vi"("Cursor No."=1.0, "Cursor"="Cursor", "3D Surface Analysis"="3D Surface") -> ("Cursor Y"=w163:dbl)  [unwired: 6 in, 2 out]
        n74 = Dequeue Element(queue=w157) -> (queue out=w156:refnum<queue>, element=w167:dbl[][])  [unwired: 2 in, 2 out]
        n75 = Add(x=0.0, y=w163) -> (x+y=w166:dbl)
        n76 = Index Array(array=w167, index (col)=w166) -> (element=→"Feature extraction scan":dbl[])  [unwired: 1 in]
        n77 = local read "Completed"() -> (w159:bool)
        n78 = local read "Exit"() -> (w155:bool)
        n79 = call <vilib>:"3D Surface.vi"("z matrix"=w167, "3D graph"="3D Surface") -> ()  [unwired: 8 in, 2 out]
        n80 = Wait Until Next ms Multiple(millisecond multiple=u32 100 ("ms 배수")) -> ()  [unwired: 1 out]
        n81 = Compound Arithmetic op=OR(w155, w159) -> (w158:bool)
      }
      n82 = Release Queue(queue=w38) -> ()  [unwired: 2 in, 3 out]
      n83 = call <vilib>:"DAQmx Stop Task.vi"("task/channels in"=w93, "error in"=w92) -> ()  [unwired: 12 in, 2 out]
      n84 = Release Queue(queue=w39) -> ()  [unwired: 2 in, 3 out]
      n85 = Release Queue(queue=w76, error in (no error)=w82) -> ()  [unwired: 1 in, 3 out]
    }
    frame True {
    }
  }
  n86 = local read "Travel per Pulse (mm)"() -> (w25:dbl)
  n87 = call-poly "VISA Configure Serial Port"("VISA resource name"="COM X", "baud rate (9600)"="Baud Rate", "data bits (8)"="Data bits", "parity (0:none)"="Parity", "stop bits (10: 1 bit)"="Stop bits", "flow control (0:none)"="Flow control") -> ("VISA resource name out"=w35:refnum<visa-resource-name>, "error out"=w34:errorcluster)  [unwired: 8 in]
  n88 = local read "Speed (mm/s)"() -> (w27:dbl)
  n89 = local read "Multiplier"() -> (w26:dbl)
  n90 = call-poly "VISA Configure Serial Port"("VISA resource name"="COM Y", "baud rate (9600)"="Baud Rate", "data bits (8)"="Data bits", "parity (0:none)"="Parity", "stop bits (10: 1 bit)"="Stop bits", "flow control (0:none)"="Flow control") -> ("VISA resource name out"=w30:refnum<visa-resource-name>, "error out"=w29:errorcluster)  [unwired: 8 in]
  n91 = call "Autonics_Speed.vi"("Multiplier"=w26, "Speed (mm/s)"=w27, "error in (no error)"=w29, "Travel per  Pulse"=w25, "VISA resource name"=w30) -> ("error out"=w15:errorcluster, "VISA resource name out"=w16:refnum<visa-resource-name>)  [unwired: 5 in]
  n92 = call "Autonics_Speed.vi"("Multiplier"="Multiplier", "Speed (mm/s)"="Speed (mm/s)", "error in (no error)"=w34, "Travel per  Pulse"="Travel per Pulse (mm)", "VISA resource name"=w35) -> ("error out"=w17:errorcluster, "VISA resource name out"=w18:refnum<visa-resource-name>)  [unwired: 5 in]
  n93 = while {
    shift-right: [w261] -> w4
    shift-left: w18 -> [w260]
    shift-right: [w251] -> w5
    shift-left: w17 -> [w259]
    shift-right: [w254] -> w3
    shift-left: w16 -> [w256]
    shift-right: [w253] -> w2
    shift-left: w15 -> [w255]
    stop <- w258 stop-if-true
    n94 = event shown="[0] Timeout" {
      selector: _ -> [_ _ _ _ _ _ _ _ _]
      dyn-events: _ -> [_ _ _ _ _ _ _ _ _]
      timeout: 100 -> [_ _ _ _ _ _ _ _ _]
      tunnel: w260 -> [w269 w291 w309 w314 w326 w346 w359 w382 w409]
      tunnel: w259 -> [w268 w290 w308 w313 w327 w345 w358 w381 w408]
      tunnel: [w265 w289 w307 w316 w326 w348 w359 w379 w411] -> w261
      tunnel: [w264 w288 w306 w315 w327 w347 w358 w378 w410] -> w251
      tunnel: [_ "Exit" _ _ _ _ _ _ _] -> w257
      tunnel: w256 -> [w267 w286 w305 w311 w331 w343 w362 w377 w406]
      tunnel: w255 -> [w266 w287 w302 w310 w330 w342 w363 w376 w404]
      tunnel: [w263 w286 w304 w311 w329 w343 w360 w374 w405] -> w254
      tunnel: [w262 w287 w303 w310 w328 w342 w361 w375 w403] -> w253
      event Timeout {
        n95 = event-data() -> ()  [unwired: 1 in, 1 out]
        n96 = local read "Scan"() -> (w270:bool)
        n97 = case shown="False" w270 {
          tunnel: w267 -> [w281 w283]
          tunnel: w266 -> [w280 w282]
          tunnel: [w279 w283] -> w263
          tunnel: [w278 w282] -> w262
          tunnel: w268 -> [w277 w284]
          tunnel: w269 -> [w276 w285]
          tunnel: [w275 w285] -> w265
          tunnel: [w274 w284] -> w264
          frame False {
            n98 = local read "Travel per Pulse (mm)"() -> (w273:dbl)
            n99 = call "Autonics_GetPos.vi"("error in (no error)"=w280, "Travel per Pulse (mm)"=w273, "VISA resource name"=w281) -> ("error out"=w278:errorcluster, "Current  Position (mm)"=w271:dbl, "VISA resource name out"=w279:refnum<visa-resource-name>)  [unwired: 6 in]
            n100 = call "Autonics_GetPos.vi"("error in (no error)"=w277, "Travel per Pulse (mm)"=w273, "VISA resource name"=w276) -> ("error out"=w274:errorcluster, "Current  Position (mm)"=w272:dbl, "VISA resource name out"=w275:refnum<visa-resource-name>)  [unwired: 6 in]
            n101 = local write "Y Current.Pos(mm)"(w271) -> ()
            n102 = local write "X Current.Pos(mm)"(w272) -> ()
          }
          frame True {
          }
        }
      }
      event "Exit": Value Change {
        n103 = event-data() -> ()  [unwired: 1 in, 5 out]
        n104 = case shown="True" "Exit" {
          tunnel: [w294 w297] -> w289
          tunnel: [w293 w298] -> w288
          tunnel: w291 -> [w294 w296]
          tunnel: w290 -> [w293 w295]
          frame False {
          }
          frame True {
            n105 = call "Autonics_Stop.vi"("error in (no error)"=w295, "VISA resource name"=w296) -> ("error out"=w298:errorcluster, "VISA resource name out"=w297:refnum<visa-resource-name>)  [unwired: 8 in]
          }
        }
      }
      event "Speed (mm/s)": Value Change {
        n106 = event-data() -> ()  [unwired: 1 in, 1 out]
        n107 = local read "Multiplier"() -> (w299:dbl)
        n108 = local read "Speed (mm/s)"() -> (w300:dbl)
        n109 = local read "Travel per Pulse (mm)"() -> (w301:dbl)
        n110 = call "Autonics_Speed.vi"("Multiplier"=w299, "Speed (mm/s)"=w300, "error in (no error)"=w308, "Travel per  Pulse"=w301, "VISA resource name"=w309) -> ("error out"=w306:errorcluster, "VISA resource name out"=w307:refnum<visa-resource-name>)  [unwired: 5 in]
        n111 = call "Autonics_Speed.vi"("Multiplier"=w299, "Speed (mm/s)"=w300, "error in (no error)"=w302, "Travel per  Pulse"=w301, "VISA resource name"=w305) -> ("error out"=w303:errorcluster, "VISA resource name out"=w304:refnum<visa-resource-name>)  [unwired: 5 in]
      }
      event "Right": Value Change {
        n112 = event-data() -> ()  [unwired: 1 in, 1 out]
        n113 = case shown="True" "Right" {
          tunnel: [w317 w323] -> w316
          tunnel: [w318 w319] -> w315
          tunnel: w314 -> [w317 w325]
          tunnel: w313 -> [w318 w324]
          frame False {
          }
          frame True {
            n114 = local read "Travel per Pulse (mm)"() -> (w321:dbl)
            n115 = local read "Move Dis(mm)"() -> (w322:dbl)
            n116 = call "Autonics_Move.vi"("Direction (+)"="-", "error in (no error)"=w324, "Travel per Pulse (mm)"=w321, "Move Distance (mm)"=w322, "VISA resource name"=w325) -> ("error out"=w319:errorcluster, "VISA resource name out"=w323:refnum<visa-resource-name>)  [unwired: 5 in]
          }
        }
      }
      event "Forward": Value Change {
        n117 = event-data() -> ()  [unwired: 1 in, 1 out]
        n118 = case shown="True" "Forward" {
          tunnel: [w333 w339] -> w329
          tunnel: [w334 w338] -> w328
          tunnel: w331 -> [w333 w341]
          tunnel: w330 -> [w334 w340]
          frame False {
          }
          frame True {
            n119 = local read "Travel per Pulse (mm)"() -> (w336:dbl)
            n120 = local read "Move Dis(mm)"() -> (w337:dbl)
            n121 = call "Autonics_Move.vi"("Direction (+)"="+", "error in (no error)"=w340, "Travel per Pulse (mm)"=w336, "Move Distance (mm)"=w337, "VISA resource name"=w341) -> ("error out"=w338:errorcluster, "VISA resource name out"=w339:refnum<visa-resource-name>)  [unwired: 5 in]
          }
        }
      }
      event "Left": Value Change {
        n122 = event-data() -> ()  [unwired: 1 in, 1 out]
        n123 = case shown="True" "Left" {
          tunnel: [w350 w355] -> w348
          tunnel: [w349 w354] -> w347
          tunnel: w346 -> [w350 w357]
          tunnel: w345 -> [w349 w356]
          frame False {
          }
          frame True {
            # "Moving distance"
            n124 = local read "Travel per Pulse (mm)"() -> (w351:dbl)
            n125 = local read "Move Dis(mm)"() -> (w352:dbl)
            n126 = call "Autonics_Move.vi"("Direction (+)"="+", "error in (no error)"=w356, "Travel per Pulse (mm)"=w351, "Move Distance (mm)"=w352, "VISA resource name"=w357) -> ("error out"=w354:errorcluster, "VISA resource name out"=w355:refnum<visa-resource-name>)  [unwired: 5 in]
          }
        }
      }
      event "Backward": Value Change {
        n127 = event-data() -> ()  [unwired: 1 in, 1 out]
        n128 = case shown="True" "Backward" {
          tunnel: [w366 w371] -> w360
          tunnel: [w365 w370] -> w361
          tunnel: w362 -> [w366 w373]
          tunnel: w363 -> [w365 w372]
          frame False {
          }
          frame True {
            # "Moving distance"
            n129 = local read "Travel per Pulse (mm)"() -> (w367:dbl)
            n130 = local read "Move Dis(mm)"() -> (w368:dbl)
            n131 = call "Autonics_Move.vi"("Direction (+)"="-", "error in (no error)"=w372, "Travel per Pulse (mm)"=w367, "Move Distance (mm)"=w368, "VISA resource name"=w373) -> ("error out"=w370:errorcluster, "VISA resource name out"=w371:refnum<visa-resource-name>)  [unwired: 5 in]
          }
        }
      }
      event "Home": Value Change {
        n132 = event-data() -> ()  [unwired: 1 in, 1 out]
        n133 = case shown="True" "Home" {
          tunnel: [w386 w398] -> w379
          tunnel: [w385 w397] -> w378
          tunnel: w382 -> [w386 w402]
          tunnel: w381 -> [w385 w401]
          tunnel: w377 -> [w384 w394]
          tunnel: w376 -> [w383 w393]
          tunnel: [w384 w392] -> w374
          tunnel: [w383 w391] -> w375
          frame False {
          }
          frame True {
            n134 = call "Autonics_Home.vi"("error in (no error)"=w401, "VISA resource name"=w402) -> ("error out"=w399:errorcluster, "VISA resource name out"=w400:refnum<visa-resource-name>)  [unwired: 8 in]
            n135 = call "Autonics_Home.vi"("error in (no error)"=w393, "VISA resource name"=w394) -> ("error out"=w396:errorcluster, "VISA resource name out"=w395:refnum<visa-resource-name>)  [unwired: 8 in]
            n136 = local read "Speed (mm/s)"() -> (w389:dbl)
            n137 = local read "Travel per Pulse (mm)"() -> (w390:dbl)
            n138 = local read "Multiplier"() -> (w388:dbl)
            n139 = local write "Home"(FALSE ("Home")) -> ()
            n140 = call "Autonics_Speed.vi"("Multiplier"=w388, "Speed (mm/s)"=w389, "error in (no error)"=w399, "Travel per  Pulse"=w390, "VISA resource name"=w400) -> ("error out"=w397:errorcluster, "VISA resource name out"=w398:refnum<visa-resource-name>)  [unwired: 5 in]
            n141 = call "Autonics_Speed.vi"("Multiplier"=w388, "Speed (mm/s)"=w389, "error in (no error)"=w396, "Travel per  Pulse"=w390, "VISA resource name"=w395) -> ("error out"=w391:errorcluster, "VISA resource name out"=w392:refnum<visa-resource-name>)  [unwired: 5 in]
          }
        }
      }
      event "Stop": Value Change {
        n142 = event-data() -> ()  [unwired: 1 in, 1 out]
        n143 = case shown="False" "Stop" {
          tunnel: [w413 w420] -> w411
          tunnel: [w415 w423] -> w410
          tunnel: w409 -> [w413 w422]
          tunnel: w408 -> [w415 w421]
          tunnel: w406 -> [w414 w419]
          tunnel: [w414 w418] -> w405
          tunnel: w404 -> [w412 w417]
          tunnel: [w412 w416] -> w403
          frame False {
          }
          frame True {
            n144 = call "Autonics_Stop.vi"("error in (no error)"=w421, "VISA resource name"=w422) -> ("error out"=w423:errorcluster, "VISA resource name out"=w420:refnum<visa-resource-name>)  [unwired: 8 in]
            n145 = call "Autonics_Stop.vi"("error in (no error)"=w417, "VISA resource name"=w419) -> ("error out"=w416:errorcluster, "VISA resource name out"=w418:refnum<visa-resource-name>)  [unwired: 8 in]
          }
        }
      }
    }
    n146 = Unbundle By Name(w253) -> ("status"=w252:bool)
    n147 = Unbundle By Name(w251) -> ("status"=w250:bool)
    n148 = Compound Arithmetic op=OR(w252, w257, w250) -> (w258:bool)
  }
  n149 = VISA Close(VISA resource name=w4, error in (no error)=w5) -> (error out=w7:errorcluster)
  n150 = VISA Close(VISA resource name=w3, error in (no error)=w2) -> (error out=w6:errorcluster)
  n151 = call <vilib>:"Simple Error Handler.vi"("error in (no error)"=w7) -> ()  [unwired: 4 in, 5 out]
  n152 = call <vilib>:"Simple Error Handler.vi"("error in (no error)"=w6) -> ()  [unwired: 4 in, 5 out]
  n153 = while {
    shift-right: [w442] -> _
    shift-left: T1."No Scan" -> [w447]
    shift-right: [w438] -> _
    shift-left: 0.0 ("Current  Position (mm)") -> [w446]
    shift-right: [w439] -> _
    shift-left: 0.0 ("Current  Position (mm)") -> [w445]
    shift-right: [w437] -> _
    shift-left: 0.0 ("Current  Position (mm)") -> [w444]
    shift-right: [w436] -> _
    shift-left: 0.0 ("Current  Position (mm)") -> [w443]
    tunnel: w17 -> [w441]
    tunnel: w18 -> [w428]
    tunnel: w15 -> [w440]
    tunnel: w16 -> [w427]
    tunnel: [w435] -> _
    tunnel: [w433] -> w9
    tunnel: [w434] -> _
    tunnel: [w432] -> w8
    shift-right: [w425] -> _
    shift-left: 0.0 ("Current  Position (mm)") -> [w424]
    stop <- w429 stop-if-true
    n154 = case shown="\"Move X\"" w447 {
      selector: w447 -> [w465 _ _ _ _]
      tunnel: w446 -> [w458 w507 w529 w593 w633]
      tunnel: w445 -> [w459 w506 w535 w592 w632]
      tunnel: w444 -> [_ w505 w552 w573 w616]
      tunnel: w443 -> [_ w504 w553 w591 w614]
      tunnel: [w464 T1."Wait X" w531 w584 w618] -> w442
      tunnel: w441 -> [w463 w499 w548 w582 w627]
      tunnel: w428 -> [w462 w500 w549 w583 w628]
      tunnel: w440 -> [w461 w501 w541 w578 w630]
      tunnel: w427 -> [w460 w502 w542 w579 w629]
      tunnel: [w451 w506 w535 w592 w632] -> w439
      tunnel: [w450 w507 w532 w593 w633] -> w438
      tunnel: [w453 w505 w552 w573 w631] -> w437
      tunnel: [w452 w504 w553 w591 w614] -> w436
      tunnel: [w457 w493 w546 w581 w625] -> w435
      tunnel: [w456 w492 w544 w580 w623] -> w433
      tunnel: [w455 w491 w550 w576 w621] -> w434
      tunnel: [w454 w490 w551 w577 w619] -> w432
      tunnel: w428 -> [_ _ _ _ _]
      tunnel: [w449 w489 w522 w571 w610] -> w425
      tunnel: w424 -> [w448 w489 w528 w571 w610]
      frame "No Scan", Default {
        n155 = case shown="False" "Scan" {
          tunnel: w465 -> [w474 _]
          tunnel: [w474 T1."Move X"] -> w464
          tunnel: w463 -> [w471 w482]
          tunnel: w462 -> [w472 w481]
          tunnel: w461 -> [w469 w480]
          tunnel: w460 -> [w470 w479]
          tunnel: w459 -> [w468 _]
          tunnel: w458 -> [w473 _]
          tunnel: [w473 w476] -> w450
          tunnel: [w472 w488] -> w457
          tunnel: [w471 w487] -> w456
          tunnel: [w470 w486] -> w455
          tunnel: [w469 w485] -> w454
          tunnel: [w468 w483] -> w453
          tunnel: [w467 w476] -> w449
          tunnel: w448 -> [w467 _]
          frame False {
          }
          frame True {
            n156 = local write "Direction (+)"("+" ("Direction (+)")) -> ()
            n157 = local write "Numeric"(0.0 ("Numeric")) -> ()
            n158 = local read "Travel per Pulse (mm)"() -> (w478:dbl)
            n159 = call "Autonics_GetPos.vi"("error in (no error)"=w482, "Travel per Pulse (mm)"=w478, "VISA resource name"=w481) -> ("error out"=w487:errorcluster, "Current  Position (mm)"=w476:dbl, "VISA resource name out"=w488:refnum<visa-resource-name>)  [unwired: 6 in]
            "Start Pos Y" <- w476
            n160 = call "Autonics_GetPos.vi"("error in (no error)"=w480, "Travel per Pulse (mm)"=w478, "VISA resource name"=w479) -> ("error out"=w485:errorcluster, "Current  Position (mm)"=w483:dbl, "VISA resource name out"=w486:refnum<visa-resource-name>)  [unwired: 6 in]
            "Start Pos X" <- w483
            n161 = local write "Y Current.Pos(mm)"(w483) -> ()
            n162 = local write "X Current.Pos(mm)"(w476) -> ()
          }
        }
        n163 = local read "X - length"() -> (w451:dbl)
        n164 = local read "Step Y"() -> (w452:dbl)
      }
      frame "Move X" {
        n165 = local read "Travel per Pulse (mm)"() -> (w494:dbl)
        n166 = local read "X - length"() -> (w495:dbl)
        n167 = call "Autonics_Move.vi"("Direction (+)"="Direction (+)", "error in (no error)"=w499, "Travel per Pulse (mm)"=w494, "Move Distance (mm)"=w495, "VISA resource name"=w500) -> ("error out"=w497:errorcluster, "VISA resource name out"=w498:refnum<visa-resource-name>)  [unwired: 5 in]
        n168 = flat-sequence {
          tunnel: [w512] -> w493
          tunnel: w498 -> [w512]
          tunnel: [w511] -> w492
          tunnel: w497 -> [w511]
          tunnel: [w509] -> w491
          tunnel: w502 -> [w509]
          tunnel: [w508] -> w490
          tunnel: w501 -> [w508]
          frame #0 {
            n169 = Wait (ms)(milliseconds to wait=u32 100) -> ()  [unwired: 1 out]
          }
        }
      }
      frame "Wait X" {
        n170 = local read "Travel per Pulse (mm)"() -> (w539:dbl)
        n171 = call "Autonics_GetPos.vi"("error in (no error)"=w541, "Travel per Pulse (mm)"=w539, "VISA resource name"=w542) -> ("error out"=w540:errorcluster, "Current  Position (mm)"=w538:dbl, "VISA resource name out"=w543:refnum<visa-resource-name>)  [unwired: 6 in]
        n172 = call "Autonics_GetPos.vi"("error in (no error)"=w548, "Travel per Pulse (mm)"=w539, "VISA resource name"=w549) -> ("error out"=w545:errorcluster, "Current  Position (mm)"=w520:dbl, "VISA resource name out"=w547:refnum<visa-resource-name>)  [unwired: 6 in]
        n173 = local write "Y Current.Pos(mm)"(w538) -> ()
        n174 = local read "Direction (+)"() -> (w515:string)
        n175 = Equal?(x=w515, y="-") -> (x = y?=w513:bool)
        n176 = local write "X Current.Pos(mm)"(w520) -> ()
        n177 = local read "Step X"() -> (w525:dbl)
        n178 = Subtract(x=w520, y=w528) -> (x-y=w527:dbl)
        n179 = Absolute Value(x=w535) -> (abs(x)=w537:dbl)
        n180 = Absolute Value(x=w527) -> (abs(x)=w526:dbl)
        n181 = Subtract(x=w520, y=w529) -> (x-y=w536:dbl)
        n182 = Greater Or Equal?(x=w526, y=w525) -> (x >= y?=w521:bool)
        n183 = Quotient & Remainder(x=w520, y=w525) -> (floor(x/y)=w517:dbl)  [unwired: 1 out]
        n184 = Absolute Value(x=w536) -> (abs(x)=w530:dbl)
        n185 = Subtract(x=w530, y=w537) -> (x-y=w533:dbl)
        n186 = case shown="True" w521 {
          selector: w521 -> [_ w554]
          frame False {
          }
          frame True {
            n187 = local read "Numeric"() -> (w556:dbl)
            n188 = Increment(x=w556) -> (x+1=→"Numeric":dbl)
            "Acquire" <- w554
          }
        }
        n189 = Increment(x=w517) -> (x+1=w518:dbl)
        n190 = call "Convert Double Precision.vi"("Input"=w533) -> ("Output"=w534:dbl)  [unwired: 10 in]
        n191 = Select(t=w518, s=w513, f=w517) -> (s? t:f=w516:dbl)
        n192 = Multiply(x=w516, y=w525) -> (x*y=w524:dbl)
        n193 = Select(t=w524, s=w521, f=w528) -> (s? t:f=w523:dbl)
        n194 = Greater Or Equal To 0?(x=w534) -> (x >= 0?=w519:bool)
        n195 = Select(t=w520, s=w519, f=w523) -> (s? t:f=w522:dbl)
        n196 = case shown="True" w519 {
          tunnel: [w559 w570] -> w551
          tunnel: w540 -> [w559 w570]
          tunnel: [w560 w569] -> w550
          tunnel: w543 -> [w560 w569]
          tunnel: [w562 w568] -> w546
          tunnel: w547 -> [w562 w568]
          tunnel: [w561 w567] -> w544
          tunnel: w545 -> [w561 w567]
          tunnel: [w558 w566] -> w532
          tunnel: w529 -> [w558 _]
          tunnel: [T1."Wait X" T1."Move Y"] -> w531
          frame False {
          }
          frame True {
            n197 = local read "X Current.Pos(mm)"() -> (w566:dbl)
            n198 = local write "Numeric"(0.0 ("Numeric")) -> ()
            n199 = Wait (ms)(milliseconds to wait=u32 1000) -> ()  [unwired: 1 out]
          }
        }
        "Current  Position (mm)" <- w528
      }
      frame "Move Y" {
        n200 = local read "Step Y"() -> (w587:dbl)
        n201 = local read "Y - length"() -> (w572:dbl)
        n202 = local read "Start Pos Y"() -> (w574:dbl)
        n203 = Subtract(x=w572, y=w587) -> ()  [unwired: 1 out]
        n204 = Subtract(x=w574, y=w573) -> (x-y=w590:dbl)
        n205 = Absolute Value(x=w572) -> (abs(x)=w588:dbl)
        n206 = Absolute Value(x=w590) -> (abs(x)=w589:dbl)
        n207 = Subtract(x=w589, y=w588) -> (x-y=w586:dbl)
        n208 = call "Convert Double Precision.vi"("Input"=w586) -> ("Output"=w585:dbl)  [unwired: 10 in]
        n209 = Greater Or Equal To 0?(x=w585) -> (x >= 0?=w575:bool)
        n210 = case shown="False" w575 {
          tunnel: [T1."Wait Y" T1."No Scan"] -> w584
          tunnel: w583 -> [w601 w607]
          tunnel: [w602 w606] -> w580
          tunnel: w582 -> [w602 w606]
          tunnel: [w601 w607] -> w581
          tunnel: w579 -> [w595 w605]
          tunnel: w578 -> [w599 w604]
          tunnel: [w600 w604] -> w577
          tunnel: [w594 w605] -> w576
          frame False {
            n211 = local read "Step Y"() -> (w598:dbl)
            n212 = local read "Travel per Pulse (mm)"() -> (w596:dbl)
            n213 = call "Autonics_Move.vi"("Direction (+)"="+" ("Direction (+) 2"), "error in (no error)"=w599, "Travel per Pulse (mm)"=w596, "Move Distance (mm)"=w598, "VISA resource name"=w595) -> ("error out"=w600:errorcluster, "VISA resource name out"=w594:refnum<visa-resource-name>)  [unwired: 5 in]
          }
          frame True {
            n214 = local write "Scan"(FALSE) -> ()
          }
        }
      }
      frame "Wait Y" {
        n215 = local read "Travel per Pulse (mm)"() -> (w611:dbl)
        n216 = call "Autonics_GetPos.vi"("error in (no error)"=w630, "Travel per Pulse (mm)"=w611, "VISA resource name"=w629) -> ("error out"=w620:errorcluster, "Current  Position (mm)"=w615:dbl, "VISA resource name out"=w622:refnum<visa-resource-name>)  [unwired: 6 in]
        n217 = call "Autonics_GetPos.vi"("error in (no error)"=w627, "Travel per Pulse (mm)"=w611, "VISA resource name"=w628) -> ("error out"=w624:errorcluster, "Current  Position (mm)"=w617:dbl, "VISA resource name out"=w626:refnum<visa-resource-name>)  [unwired: 6 in]
        n218 = Subtract(x=w615, y=w616) -> (x-y=w635:dbl)
        n219 = Absolute Value(x=w614) -> (abs(x)=w637:dbl)
        n220 = Absolute Value(x=w635) -> (abs(x)=w636:dbl)
        n221 = local write "Y Current.Pos(mm)"(w615) -> ()
        n222 = local write "X Current.Pos(mm)"(w617) -> ()
        n223 = Subtract(x=w636, y=w637) -> (x-y=w634:dbl)
        n224 = call "Convert Double Precision.vi"("Input"=w634) -> ("Output"=w613:dbl)  [unwired: 10 in]
        n225 = Greater Or Equal To 0?(x=w613) -> (x >= 0?=w612:bool)
        n226 = case shown="True" w612 {
          tunnel: w616 -> [w643 _]
          tunnel: [w643 w656] -> w631
          tunnel: w626 -> [w642 w654]
          tunnel: [w642 w654] -> w625
          tunnel: [w641 w653] -> w623
          tunnel: w624 -> [w641 w653]
          tunnel: [w640 w652] -> w621
          tunnel: w622 -> [w640 w652]
          tunnel: [w639 w651] -> w619
          tunnel: w620 -> [w639 w651]
          tunnel: [T1."Wait Y" T1."Move X"] -> w618
          frame False {
          }
          frame True {
            n227 = local read "Y Current.Pos(mm)"() -> (w656:dbl)
            n228 = local read "Direction (+)"() -> (w650:string)
            n229 = Equal?(x=w650, y="+") -> (x = y?=w648:bool)
            n230 = Select(t="-", s=w648, f="+") -> (s? t:f=w647:string)
            n231 = local write "Direction (+)"(w647) -> ()
            n232 = Wait (ms)(milliseconds to wait=u32 1000) -> ()  [unwired: 1 out]
          }
        }
      }
    }
    n233 = Wait Until Next ms Multiple(millisecond multiple=u32 100 ("milliseconds to wait")) -> ()  [unwired: 1 out]
    n234 = Unbundle By Name(w433) -> ("status"=w431:bool)
    n235 = Unbundle By Name(w432) -> ("status"=w430:bool)
    n236 = Compound Arithmetic op=OR(w431, w430) -> (w429:bool)
    "Enum" <- w447
  }
  n237 = call <vilib>:"Simple Error Handler.vi"("error in (no error)"=w9) -> ()  [unwired: 4 in, 5 out]
  n238 = call <vilib>:"Simple Error Handler.vi"("error in (no error)"=w8) -> ()  [unwired: 4 in, 5 out]
